vi "Find Controllers 2.vi"(8 "error in (no error)":errorcluster, 10 "Numeric":u32) -> (0 "error out":errorcluster, 2 "Names":string[](array[string]))   [LabVIEW 2020]
uses:
  libximc.lvlib
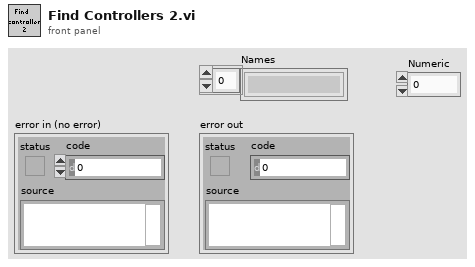
[diagram p1: front panel]
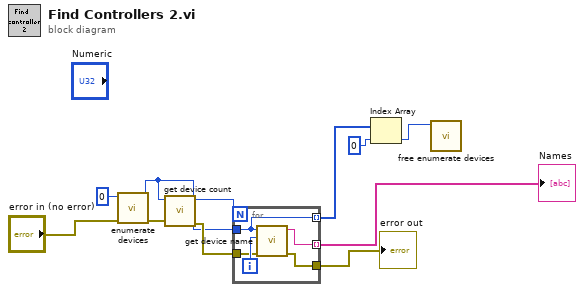
[diagram p0: block diagram]
diagram:
  n1 = call "enumerate devices.vi"("error in (no error)"="error in (no error)", "enumerate_flags"=0 ("probe_devices")) -> ("error out"=w7:errorcluster, "function return"=w4:u32)  [unwired: 8 in]
  n2 = call "get device count.vi"("error in (no error)"=w7, "device_enumeration"=w4) -> ("error out"=w8:errorcluster, "function return"=w9:i32)  [unwired: 8 in]
  n3 = for {
    N: w9 -> [_]
    tunnel: [w16] -> w6
    tunnel: [w15] -> w5 mode=indexing
    tunnel: w4 -> [w12]
    tunnel: w8 -> [w13]
    tunnel: [w12] -> w3 mode=indexing
    i -> [w14]
    n4 = call "get device name.vi"("error in (no error)"=w13, "device_index"=w14, "device_enumeration"=w12) -> ("error out"=w16:errorcluster, "function return"=w15:string)  [unwired: 7 in]
  }
  "error out" <- w6
  "Names" <- w5
  n5 = Index Array(array=w3, index=0 ("probe_devices")) -> (element=w1:u32)
  n6 = call "free enumerate devices.vi"("device_enumeration"=w1) -> ()  [unwired: 9 in, 2 out]
